vi "WaveformAveraging.vi"(7 "NumOfWaveformsToAverage":i32=3, 10 "Array Input":dbl[](array[numeric])) -> (2 "Average N Waveforms":dbl[](array[numeric]), 6 "Averaged Waveforms":i32)   [LabVIEW 2010]
uses:
  <vilib>/Analysis/NI_AALBase.lvlib
  <vilib>/Analysis/baseanly.llb/Mean (DBL).vi
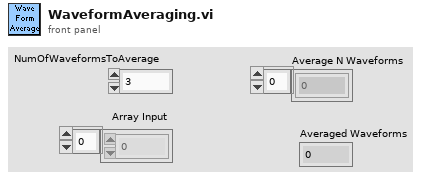
[diagram p1: front panel]
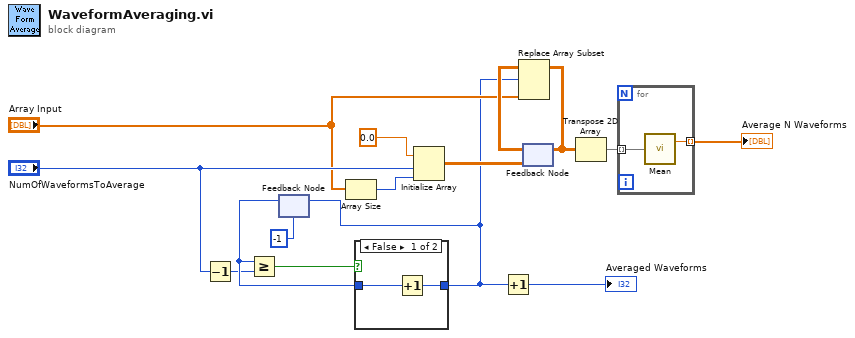
[diagram p0: block diagram]
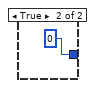
[diagram p2: hidden frame]
diagram:
  n1 = Decrement(x="NumOfWaveformsToAverage") -> (x-1=w12:i32)
  n2 = feedback #1(-1) -> (w13:i32)
  n3 = Greater Or Equal?(x=w13, y=w12) -> (x >= y?=w15:bool)
  n4 = Array Size(array="Array Input") -> (size(s)=w5:i32)
  n5 = case shown="False" w15 {
    tunnel: w13 -> [w17 _]
    tunnel: [w16 0 ("Number of waveforms to average")] -> w2
    frame False {
      n6 = Increment(x=w17) -> (x+1=w16:i32)
    }
    frame True {
    }
  }
  n7 = feedback-in #1(w2) -> ()
  n8 = Initialize Array(0.0 ("element"), "NumOfWaveformsToAverage", w5) -> (w8:dbl[][])
  n9 = Increment(x=w2) -> (x+1=→"Averaged Waveforms":i32)
  n10 = feedback #2(w8) -> (w11:dbl[][])
  n11 = Replace Array Subset(array=w11, new element="Array Input", index (row)=w2) -> (w6:dbl[][])  [unwired: 1 in]
  n12 = feedback-in #2(w6) -> ()
  n13 = Transpose 2D Array(2D array=w6) -> (transposed array=w7:dbl[][])
  n14 = for {
    tunnel: [w20] -> w3 mode=indexing
    tunnel: w7 -> [w19] mode=indexing
    n15 = call-poly <vilib>:"Mean.vi"("X"=w19) -> ("mean"=w20:dbl)  [unwired: 1 out]
  }
  "Average N Waveforms" <- w3
